vi "Log.vi"(8 "error in":errorcluster, 11 "SDO Transfer in":refnum<class "SDO Transfer.lvclass">) -> (0 "error out":errorcluster, 3 "SDO Transfer out":refnum<class "SDO Transfer.lvclass">)   [LabVIEW 2020, in "SDO Manager.lvlib" / "SDO Transfer.lvclass"]
uses:
  SDO Transfer.lvclass
  SDO Transfer.lvclass/SDO Transfer.ctl
  Logging/Log Level.vi
  Logging/CANopen Logging.lvlib
  Logging/Trace Type.ctl
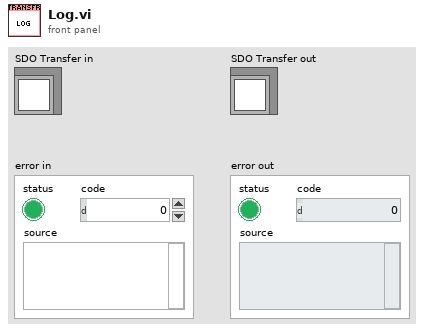
[diagram p1: front panel]
types:
  T1 = enum16{"Error", "Warn", "Info", "Debug", "Trace"}
  T2 = typedef "CANopen Logging.lvlib/Trace Type.ctl" = enum16{"Undefined", "Sent", "Received", "SDO Transfer"}
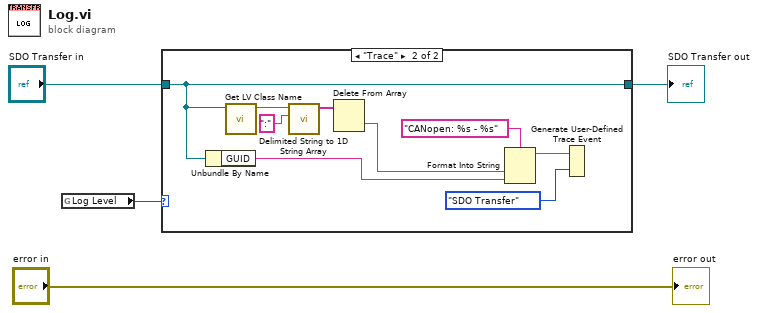
[diagram p0: block diagram]
diagram:
  n1 = global read "Log Level.vi" "Log Level"() -> (w3:T1)
  n2 = case shown="\"Trace\"" w3 {
    tunnel: "SDO Transfer in" -> [w5 w11]
    tunnel: [w5 w11] -> w4
    frame Default {
    }
    frame "Trace" {
      n3 = Unbundle By Name(w11) -> ("GUID"=w9:string)
      n4 = call <vilib>:"Get LV Class Name.vi"("object"=w11) -> ("class name"=w14:string)  [unwired: 9 in, 1 out]
      n5 = call <vilib>:"Delimited String to 1D String Array.vi"("delimiter"=":", "delimited string"=w14) -> ("string array"=w13:string[])  [unwired: 9 in]
      n6 = Delete From Array(array=w13) -> (deleted portion=w10:string)  [unwired: 2 in, 1 out]
      n7 = Format Into String(format string="CANopen: %s - %s", w10, w9) -> (resulting string=w8:string)  [unwired: 2 in, 1 out]
      n8 = Generate User-Defined Trace Event(1:Trace_Type."SDO Transfer" ("Trace Type"), 2:w8) -> ()
    }
  }
  "SDO Transfer out" <- w4
  "error out" <- "error in"
